vi "Ejemplo.vi"() -> ()   [LabVIEW 2020]
uses:
  <vilib>/ErrorRing/Error Ring.xnode
panel:
  in  "Formato":string(combo)
  in  "Nombre Archivo":string
  in  "Direccion":path
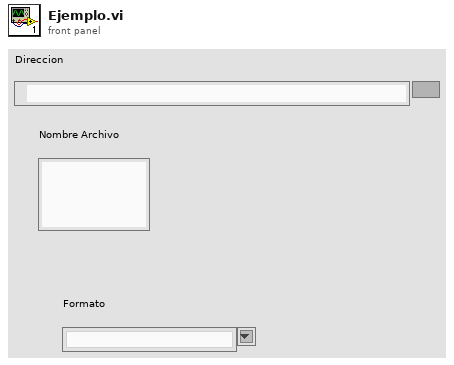
[diagram p1: front panel]
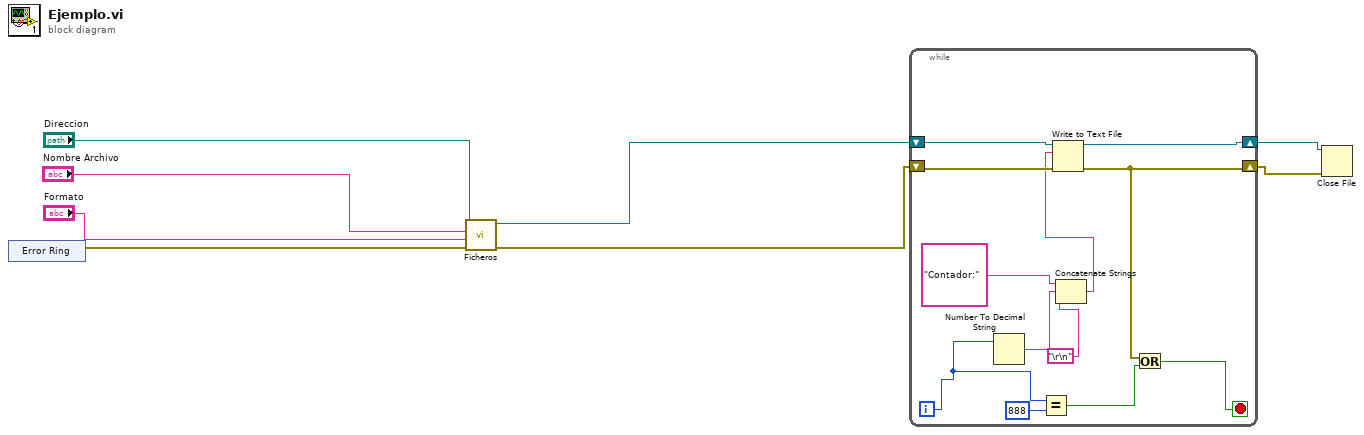
[diagram p0: block diagram]
diagram:
  n1 = xnode "Error Ring"() -> ("error out"=w5:errorcluster)
  n2 = call "Ficheros.vi"("error in (no error)"=w5, "Formato"="Formato", "Nombre Archivo"="Nombre Archivo", "Direccion"="Direccion") -> ("error out"=w1:errorcluster, "Byte Stream File out"=w2:refnum<file>)  [unwired: 6 in]
  n3 = while {
    shift-right: [w18] -> w4
    shift-left: w2 -> [w20]
    shift-right: [w10] -> w3
    shift-left: w1 -> [w19]
    i -> [w13]
    stop <- w9 stop-if-true
    n4 = Number To Decimal String(number=w13) -> (decimal integer string=w16:string)  [unwired: 1 in]
    n5 = Equal?(x=w13, y=888) -> (x = y?=w11:bool)
    n6 = Concatenate Strings("Contador:", w16, "\r\n") -> (w14:string)
    n7 = Write to Text File(file (use dialog)=w20, text=w14, error in=w19) -> (refnum out=w18:refnum<file>, error out=w10:errorcluster)  [unwired: 1 in, 1 out]
    n8 = Or(x=w10, y=w11) -> (x .or. y?=w9:bool)
  }
  n9 = Close File(refnum=w4, error in=w3) -> ()  [unwired: 2 out]
